vi "Lab2 Band Selector.vi"(10 "resistor":dbl) -> (0 "band3":dbl, 1 "band2":dbl, 2 "band1":dbl)   [LabVIEW 2016]
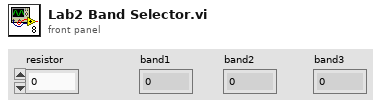
[diagram p1: front panel]
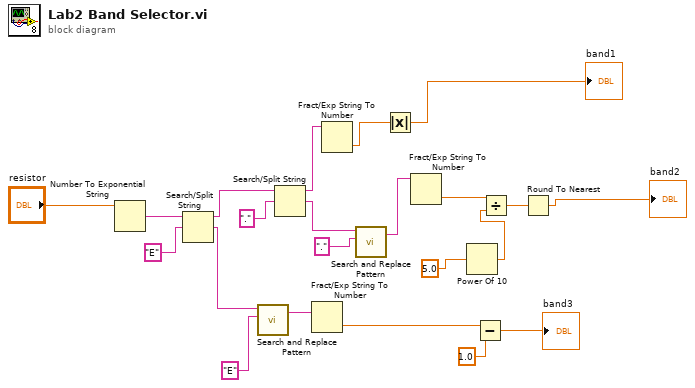
[diagram p0: block diagram]
diagram:
  n1 = Number To Exponential String(number="resistor") -> (E-format string=w21:string)  [unwired: 3 in]
  n2 = Search/Split String(string=w21, search string/char (-)="E") -> (substring before match=w15:string, match + rest of string=w17:string)  [unwired: 1 in, 1 out]
  n3 = call <vilib>:"Search and Replace Pattern.vi"("string"=w17, "regular expression (\"\")"="E") -> ("result string"=w18:string)  [unwired: 3 in, 1 out]
  n4 = Search/Split String(string=w15, search string/char (-)=".") -> (substring before match=w13:string, match + rest of string=w12:string)  [unwired: 1 in, 1 out]
  n5 = Fract/Exp String To Number(string=w18) -> (number=w8:dbl)  [unwired: 3 in, 1 out]
  n6 = Fract/Exp String To Number(string=w13) -> (number=w3:dbl)  [unwired: 3 in, 1 out]
  n7 = call <vilib>:"Search and Replace Pattern.vi"("string"=w12, "regular expression (\"\")"=".") -> ("result string"=w10:string)  [unwired: 3 in, 1 out]
  n8 = Absolute Value(x=w3) -> (abs(x)=→"band1":dbl)
  n9 = Fract/Exp String To Number(string=w10) -> (number=w5:dbl)  [unwired: 3 in, 1 out]
  n10 = Power Of 10(x=5.0) -> (10^x=w6:dbl)
  n11 = Subtract(x=w8, y=1.0) -> (x-y=→"band3":dbl)
  n12 = Divide(x=w5, y=w6) -> (x/y=w2:dbl)
  n13 = Round To Nearest(number=w2) -> (nearest integer value=→"band2":dbl)
